vi "Editor for Type.vi"(8 "Value Type String":string, 9 "Value Name":string, 10 "Is Variant":bool, 11 "Worker/Variant Folder":path) -> (0 "error out":errorcluster, 3 "Value Editor":refnum<class "Value Editor Base.lvclass">)   [LabVIEW 2020, in "FlexBlocks.lvlib"]
uses:
  FlexBlocks.lvlib
  Value Editor Base/Value Editor Base.lvclass
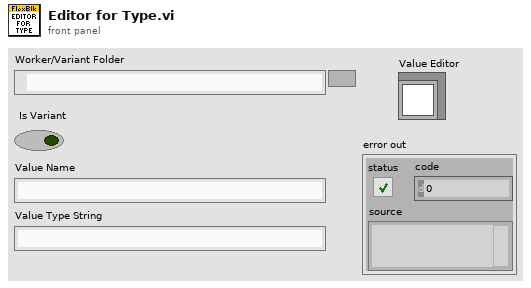
[diagram p1: front panel]
types:
  T1 = typedef "FlexBlocks.lvlib/Paths.ctl" = cluster{"FlexBlocks":path, "Workers Root":path, "Specialized Editors":path, "Worker Template":path, "Editor Template":path, "Express Template":path}
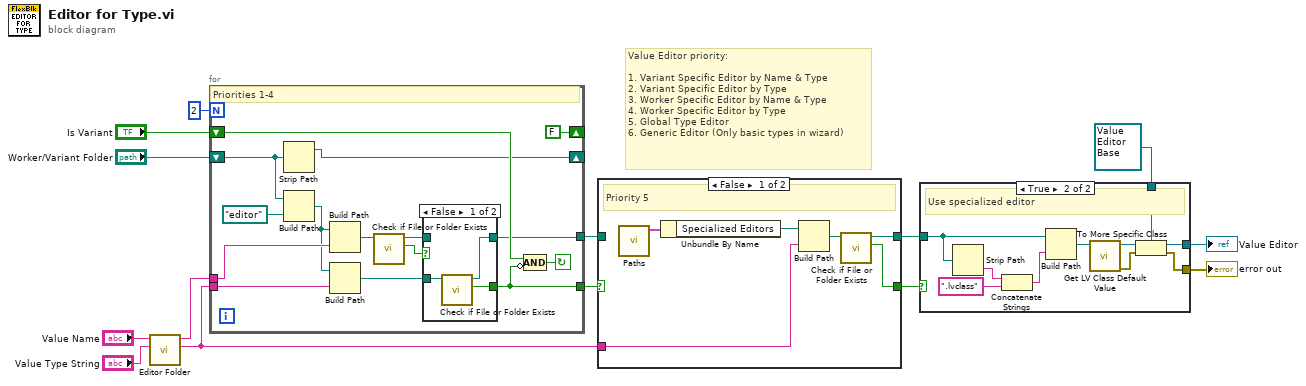
[diagram p0: block diagram]
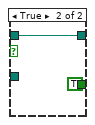
[diagram p4: hidden frame]
diagram:
  # "Value Editor priority:\n\n1. Variant Specific Editor by Name & Type\n2. Variant Specific Editor by Type\n3. Worker Specific Editor by Name & Type\n4. Worker Specific Editor by Type\n5. Global Type Editor\n6. Generic Editor (Only basic types in wizard)"
  n1 = call "Editor Folder.vi"("Value Type String"="Value Type String", "Value Name"="Value Name") -> ("Type Only Folder"=w4:string, "Name & Type Folder"=w9:string)  [unwired: 8 in]
  n2 = for {
    N: 2 -> [_]
    shift-right: [w24] -> _
    shift-left: "Worker/Variant Folder" -> [w25]
    shift-right: [FALSE ("Is Variant")] -> _
    shift-left: "Is Variant" -> [w27]
    tunnel: w9 -> [w23]
    tunnel: w4 -> [w20]
    tunnel: [w16] -> w8
    tunnel: [w15] -> w7
    stop <- w26 continue-if-true
    # "Priorities 1-4"
    n3 = Strip Path(path=w25) -> (stripped path=w24:path)  [unwired: 1 out]
    n4 = Build Path(base path=w25, name or relative path=path "editor") -> (appended path=w21:path)
    n5 = Build Path(base path=w21, name or relative path=w23) -> (appended path=w22:path)
    n6 = Build Path(base path=w21, name or relative path=w20) -> (appended path=w19:path)
    n7 = call <vilib>:"Check if File or Folder Exists.vi"("path"=w22) -> ("file or folder exists?"=w18:bool, "dup path"=w17:path)  [unwired: 8 in, 1 out]
    n8 = case shown="False" w18 {
      tunnel: w19 -> [w32 _]
      tunnel: w17 -> [_ w34]
      tunnel: [w31 TRUE ("file or folder exists?")] -> w15
      tunnel: [w30 w34] -> w16
      frame False {
        n9 = call <vilib>:"Check if File or Folder Exists.vi"("path"=w32) -> ("file or folder exists?"=w31:bool, "dup path"=w30:path)  [unwired: 8 in, 1 out]
      }
      frame True {
      }
    }
    n10 = Compound Arithmetic op=AND(w27, invert w15) -> (w26:bool)
  }
  n11 = case shown="False" w7 {
    selector: w7 -> [_ w41]
    tunnel: w8 -> [_ w42]
    tunnel: [w36 w42] -> w3
    tunnel: w4 -> [w38 _]
    tunnel: [w35 w41] -> w2
    frame False {
      # "Priority 5"
      n12 = call "Paths.vi"() -> ("Paths"=w40:T1)  [unwired: 11 in]
      n13 = Unbundle By Name(w40) -> ("Specialized Editors"=w39:path)
      n14 = Build Path(base path=w39, name or relative path=w38) -> (appended path=w37:path)
      n15 = call <vilib>:"Check if File or Folder Exists.vi"("path"=w37) -> ("file or folder exists?"=w35:bool, "dup path"=w36:path)  [unwired: 8 in, 1 out]
    }
    frame True {
      # "Editor found in 1-4"
    }
  }
  n16 = case shown="True" w2 {
    tunnel: [w43 w49] -> w6
    tunnel: [_ w47] -> w5
    tunnel: w3 -> [_ w45]
    tunnel: refnum<class "Value Editor Base.lvclass"> refnum ("Value Editor") -> [w43 w44]
    frame False {
      # "Priority 6 - Use Generic Editor"
    }
    frame True {
      # "Use specialized editor"
      n17 = Strip Path(path=w45) -> (name=w53:string)  [unwired: 1 out]
      n18 = Concatenate Strings(w53, ".lvclass" ("string")) -> (w51:string)
      n19 = Build Path(base path=w45, name or relative path=w51) -> (appended path=w50:path)
      n20 = call <vilib>:"Get LV Class Default Value.vi"("class path"=w50) -> ("error out"=w46:errorcluster, "object"=w48:refnum<class>)  [unwired: 9 in]
      n21 = To More Specific Class(target class=w44, reference=w48, error in=w46) -> (specific class reference=w49:refnum<class "Value Editor Base.lvclass">, error out=w47:errorcluster)
    }
  }
  "Value Editor" <- w6
  "error out" <- w5
